vi "Analysator duplizieren.vi"(8 "error in (no error)":errorcluster caption="Fehler (Eingang, kein Fehler)", 11 "Kombinationsfeld (Eingang)":refnum<vi>) -> (0 "error out":errorcluster caption="Fehler (Ausgang)", 3 "Strings And Values[]":T1)   [LabVIEW 2020, in "System Einstellungen V2.lvlib"]
uses:
  System Einstellungen V2.lvlib
  <vilib>/Utility/miscctls.llb/LVComboBoxStrsAndValuesArrayTypeDef.ctl
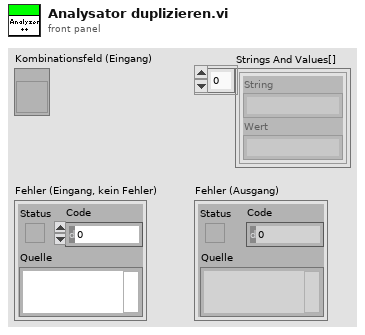
[diagram p1: front panel]
types:
  T1 = typedef "LVComboBoxStrsAndValuesArrayTypeDef.ctl" = cluster{"String":string, "Value":string}[]
  T2 = typedef "System Einstellungen V2.lvlib/Analysatoren.ctl" = string
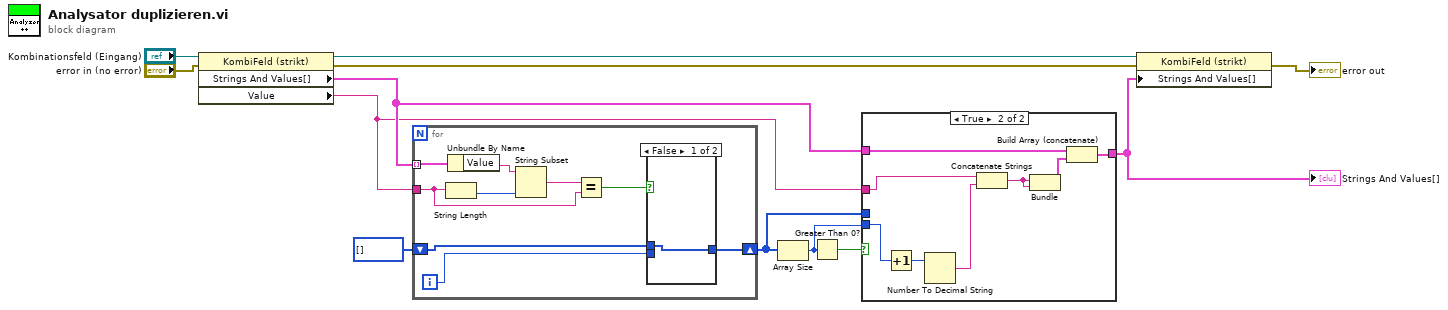
[diagram p0: block diagram]
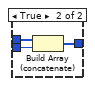
[diagram p3: hidden frame]
diagram:
  n1 = property class="KombiFeld (strikt)"(reference="Kombinationsfeld (Eingang)", error in="error in (no error)") -> (reference out=w9:refnum<vi>, error out=w10:errorcluster, "Strings And Values[]"=w6:T1, "Value"=w3:T2)
  n2 = for {
    tunnel: w6 -> [w21] mode=indexing
    tunnel: w3 -> [w17]
    shift-right: [w15] -> w4
    shift-left: i32[] [] -> [w14]
    i -> [w16]
    n3 = String Length(string=w17) -> (length=w19:i32)
    n4 = Unbundle By Name(w21) -> ("Value"=w20:string)
    n5 = String Subset(string=w20, length (rest)=w19) -> (substring=w18:string)  [unwired: 1 in]
    n6 = Equal?(x=w18, y=w17) -> (x = y?=w13:bool)
    n7 = case shown="False" w13 {
      tunnel: w16 -> [_ w25]
      tunnel: [w22 w24] -> w15
      tunnel: w14 -> [w22 w23]
      frame False {
      }
      frame True {
        n8 = Build Array (concatenate)(w23, w25) -> (w24:i32[])
      }
    }
  }
  n9 = Array Size(array=w4) -> (size(s)=w2:i32)
  n10 = Greater Than 0?(x=w2) -> (x > 0?=w5:bool)
  n11 = case shown="True" w5 {
    tunnel: w6 -> [w26 w34]
    tunnel: w4 -> [_ _]
    tunnel: w3 -> [_ w30]
    tunnel: w2 -> [_ w32]
    tunnel: [w26 w33] -> w1
    frame False {
    }
    frame True {
      n12 = Increment(x=w32) -> (x+1=w31:i32)
      n13 = Number To Decimal String(number=w31) -> (decimal integer string=w29:string)  [unwired: 1 in]
      n14 = Concatenate Strings(w30, w29) -> (w28:string)
      n15 = Bundle(w28, w28) -> (w27:cluster{string, string})  [unwired: 1 in]
      n16 = Build Array (concatenate)(w34, w27) -> (w33:T1)
    }
  }
  "Strings And Values[]" <- w1
  n17 = property class="KombiFeld (strikt)"(reference=w9, error in=w10, "Strings And Values[]"=w1) -> (error out=→"error out":errorcluster)  [unwired: 1 out]
